vi "Configure Multi Eval Meas Modulation.vi"(7 "Statistic Count (20)":i32=20, 8 "error in (no error)":errorcluster, 9 "Modulation Enabled (On)":bool=TRUE, 10 "Instance (1)":T1=1, 11 "VISA resource name":refnum<visa-resource-name>) -> (0 "error out":errorcluster, 3 "VISA resource name out":refnum<visa-resource-name>)   [LabVIEW 2015, in "Rohde&Schwarz CMXP NR FR2 Measurement.lvlib"]
doc: "Enables or disables the evaluation of modulation results in the multi-evaluation measurement.\n\nAttributes:\nRSCMXPNRFR2M_ATTR_MULTI_EVAL_MEASUREMENT_MODULATION_ENABLED\nRSCMXPNRFR2M_ATTR_MULTI_EVAL_MEASUREMENT_MODULATION_STATISTIC_COUNT\n\nRemote-control commands:\nCONFigure:NRMMw:MEAS<i>:MEValuation:RESult:MODulation\nCONFigure:NRMMw:MEAS<i>:MEValuation:SCOunt:MODulation"
uses:
  <instrlib>/Rohde&Schwarz CMXP NR FR2 Measurement/Rohde&Schwarz CMXP NR FR2 Measurement.lvlib
  <instrlib>/Rohde&Schwarz CMXP NR FR2 Measurement/Private/_Instance.ctl
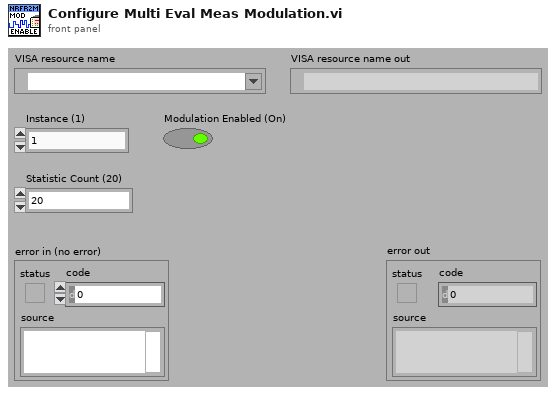
[diagram p1: front panel]
types:
  T1 = typedef "Rohde&Schwarz CMXP NR FR2 Measurement.lvlib/_Instance.ctl" = i32
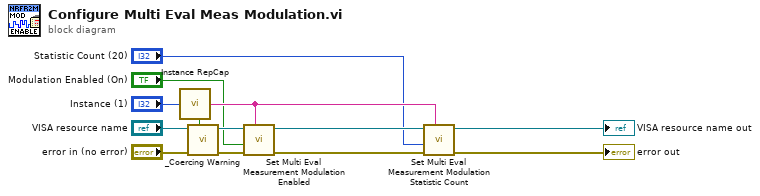
[diagram p0: block diagram]
diagram:
  n1 = call <instrlib>:"Instance RepCap.vi"("Instance In"="Instance (1)") -> ("In Range?"=w11:bool, "RepCap Identifier Out"=w6:string)  [unwired: 1 in]
  n2 = call <instrlib>:"_Coercing Warning.vi"("In Range?"=w11, "error in (no error)"="error in (no error)", "VISA resource name"="VISA resource name") -> ("error out"=w9:errorcluster, "VISA resource name out"=w10:refnum<visa-resource-name>)  [unwired: 7 in]
  n3 = call "Set Multi Eval Measurement Modulation Enabled"("Repeated Capabilities"=w6, "error in (no error)"=w9, "Multi Eval Measurement Modulation Enabled (OFF)"="Modulation Enabled (On)", "instrument handle"=w10) -> ("error out"=w4:errorcluster, "instrument handle out"=w5:refnum<visa-resource-name>)  [unwired: 6 in]
  n4 = call "Set Multi Eval Measurement Modulation Statistic Count"("Repeated Capabilities"=w6, "error in (no error)"=w4, "Multi Eval Measurement Modulation Statistic Count (0)"="Statistic Count (20)", "instrument handle"=w5) -> ("error out"=→"error out":errorcluster, "instrument handle out"=→"VISA resource name out":refnum<visa-resource-name>)  [unwired: 6 in]
